vi "System-Plot.vi"   [LabVIEW 2016, in "DSI-RT.lvlib"]
uses:
  DSI-RT.lvlib
  <vilib>/addons/Software Calibration Management/xSCM/Controls/CalPoint - Type.ctl
  <vilib>/addons/Software Calibration Management/xSCM/Get/Get Variant.vi
  <vilib>/addons/Software Calibration Management/xSCM/CalPoint-Data.vi
  <vilib>/addons/Software Calibration Management/xSCM/CalPoint.xnode
  <vilib>/addons/Software Calibration Management/xSCM/SCM-API.lvlib
  <vilib>/addons/Software Calibration Management/xSCM/ni_scm.dll
types:
  T1 = typedef "SCM-API.lvlib/CalPoint - Type.ctl" = enum8{"BOL", "U8", "U16", "U32", "U64", "I8", "I16", "I32", "I64", "SGL", "DBL", "EXT", "CSG", "CDB", "CXT", "STR", "TBL", "TLU", "CTM"}
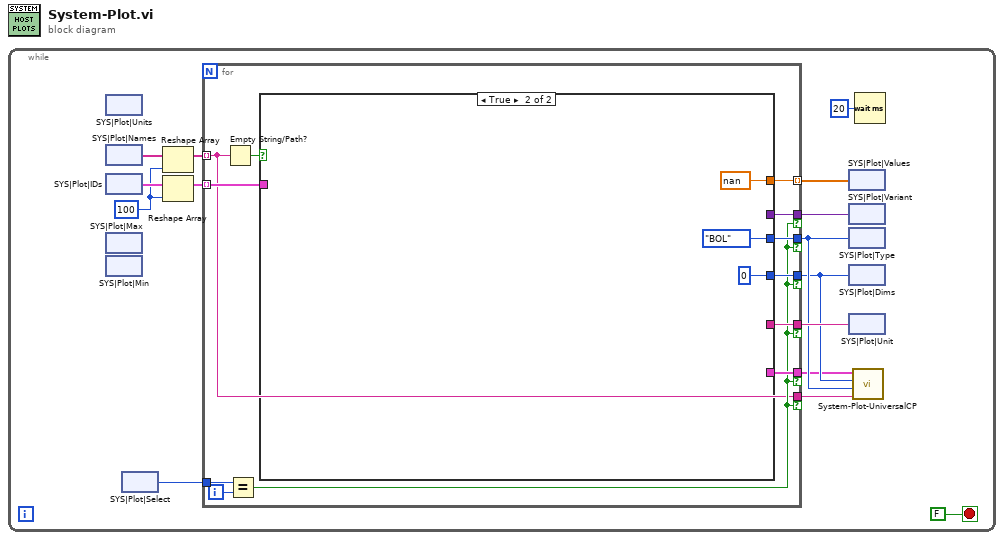
[diagram p0: block diagram]
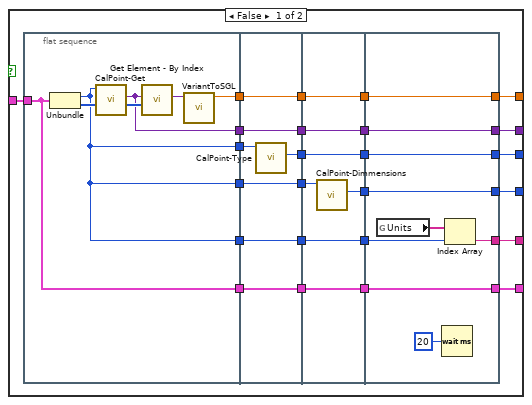
[diagram p2: hidden frame]
diagram:
  n1 = while {
    stop <- FALSE stop-if-true
    w1 = 100 ("dimension size")
    n2 = xnode "SYS|Plot|Units"() -> ()  [unwired: 1 out]
    n3 = xnode "SYS|Plot|Names"() -> ("Value"=w11:string[])
    n4 = xnode "SYS|Plot|IDs"() -> ("Value"=w12:cluster{"ID":u32, "Element":i32[]}[])
    n5 = xnode "SYS|Plot|Max"() -> ()  [unwired: 1 out]
    n6 = xnode "SYS|Plot|Min"() -> ()  [unwired: 1 out]
    n7 = xnode "SYS|Plot|Select"() -> ("Value"=w5:u8)
    n8 = Reshape Array(w11, w1) -> (w2:string[])
    n9 = Reshape Array(w12, w1) -> (w3:cluster{"ID":u32, "Element":i32[]}[])
    n10 = for {
      tunnel: [w27] -> w13 mode=indexing
      tunnel: w3 -> [w26] mode=indexing
      tunnel: w2 -> [w16] mode=indexing
      tunnel: [w25] -> w8 if=w17
      tunnel: [w24] -> w7 if=w17
      tunnel: [w23] -> w10 if=w17
      tunnel: w5 -> [w21]
      tunnel: [w20] -> w9 if=w17
      tunnel: [w19] -> w6 if=w17
      tunnel: [w16] -> w4 if=w17
      i -> [w22]
      n11 = Empty String/Path?(string/path=w16) -> (empty?=w18:bool)
      n12 = Equal?(x=w21, y=w22) -> (x = y?=w17:bool)
      n13 = case shown="True" w18 {
        tunnel: [w51 sgl nan ("Value")] -> w27
        tunnel: w26 -> [w52 _]
        tunnel: [w47 CalPoint_-_Type."BOL" ("Type")] -> w25
        tunnel: [w48 u8 0 ("Dimmensions")] -> w24
        tunnel: [w50 _] -> w23
        tunnel: [w49 _] -> w20
        tunnel: [w28 _] -> w19
        frame False {
          n14 = flat-sequence {
            tunnel: w52 -> [w55]
            tunnel: [w53] -> w46
            tunnel: [w57] -> w45
            tunnel: [w56] -> w44
            tunnel: [w56] -> w43
            tunnel: [w56] -> w42
            tunnel: [w55] -> w31
            tunnel: w46 -> [w65]
            tunnel: w45 -> [w64]
            tunnel: w44 -> [w63]
            tunnel: w43 -> [w62]
            tunnel: w42 -> [w61]
            tunnel: [w65] -> w41
            tunnel: [w64] -> w40
            tunnel: [w63] -> w39
            tunnel: [w62] -> w38
            tunnel: [w60] -> w37
            tunnel: w31 -> [w59]
            tunnel: [w59] -> w29
            tunnel: w41 -> [w72]
            tunnel: w40 -> [w71]
            tunnel: w39 -> [w70]
            tunnel: w38 -> [w68]
            tunnel: w37 -> [w69]
            tunnel: [w72] -> w36
            tunnel: [w71] -> w35
            tunnel: [w70] -> w34
            tunnel: [w67] -> w33
            tunnel: [w69] -> w32
            tunnel: [w66] -> w30
            tunnel: w29 -> [w66]
            tunnel: [w77] -> w47
            tunnel: [w78] -> w48
            tunnel: [w79] -> w49
            tunnel: [w80] -> w50
            tunnel: [w81] -> w51
            tunnel: w32 -> [w77]
            tunnel: w33 -> [w78]
            tunnel: w34 -> [w75]
            tunnel: w35 -> [w80]
            tunnel: w36 -> [w81]
            tunnel: [w73] -> w28
            tunnel: w30 -> [w73]
            frame #0 {
              n15 = Unbundle(w55) -> ("ID"=w56:u32, "Element"=w58:i32[])
              n16 = call-poly <vilib>:"CalPoint-Get.vi"("ID"=w56) -> ("Data"=w57:variant)  [unwired: 10 in]
              n17 = call <vilib>:"Get Element - By Index.vi"("Elements"=w58, "Variant"=w57) -> ("Element"=w54:variant)  [unwired: 8 in, 1 out]
              n18 = call "VariantToSGL.vi"("Element"=w54) -> ("Numeric"=w53:sgl)  [unwired: 10 in]
            }
            frame #1 {
              n19 = call <vilib>:"CalPoint-Type.vi"("ID"=w61) -> ("Type"=w60:T1)  [unwired: 10 in]
            }
            frame #2 {
              n20 = call <vilib>:"CalPoint-Dimmensions.vi"("ID"=w68) -> ("Dimmensions"=w67:u8)  [unwired: 10 in]
            }
            frame #3 {
              n21 = global read "CalPoint-Data.vi" "Units"() -> (w76:string[])
              n22 = Wait (ms)(milliseconds to wait=u32 20) -> ()  [unwired: 1 out]
              n23 = Index Array(array=w76, index=w75) -> (element=w79:string)
            }
          }
        }
        frame True {
        }
      }
    }
    n24 = xnode "SYS|Plot|Values"("Value"=w13) -> ()
    n25 = xnode "SYS|Plot|Variant"("Value"=w10) -> ()
    n26 = xnode "SYS|Plot|Type"("Value"=w8) -> ()
    n27 = xnode "SYS|Plot|Dims"("Value"=w7) -> ()
    n28 = xnode "SYS|Plot|Unit"("Value"=w9) -> ()
    n29 = call "System-Plot-UniversalCP.vi"("Name"=w4, "Type"=w8, "Dimensions"=w7, "ID"=w6) -> ()  [unwired: 8 in]
    n30 = Wait (ms)(milliseconds to wait=u32 20 ("millisecond multiple")) -> ()  [unwired: 1 out]
  }
